vi "Variable@LInsert__Parameter.vi"(1 "ParamterIn":string) -> (0 "ParamterOut":string)   [LabVIEW 2019]
uses:
  <vilib>/regexp/Match Regular Expression.xnode
panel:
  in  "Pattern":string(combo)
  in  "Before/After":string(combo)
  in  "Section":string(combo)
  in  "Value":string(combo)
  in  "Variale":string(combo)
  in  "Confirm":bool
  # "Variable@LInsert $Variable,$Value,Before|After [value1,value2...](,$Section)"
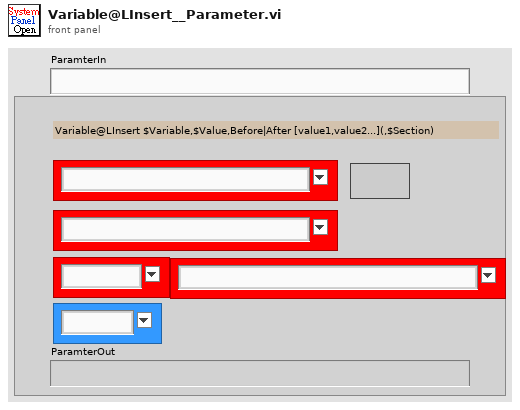
[diagram p1: front panel]
types:
  T1 = enum16{"Get", "Init", "Set", "Delete", "GetElement", "Inc", "Dec", "ReName"}
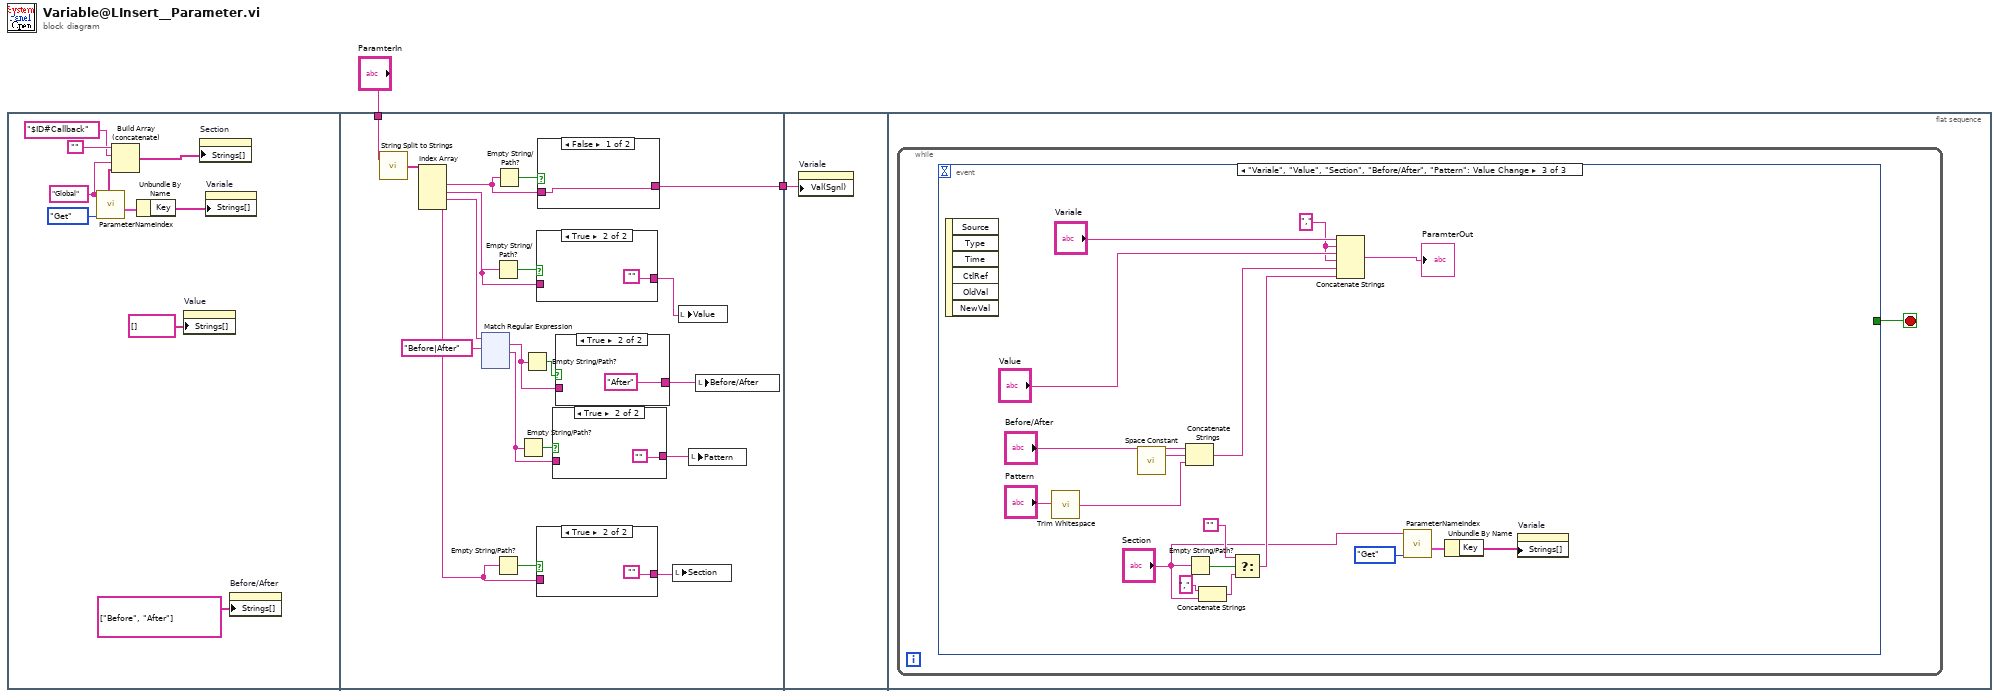
[diagram p0: block diagram]
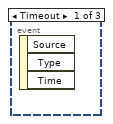
[diagram p7: hidden frame]
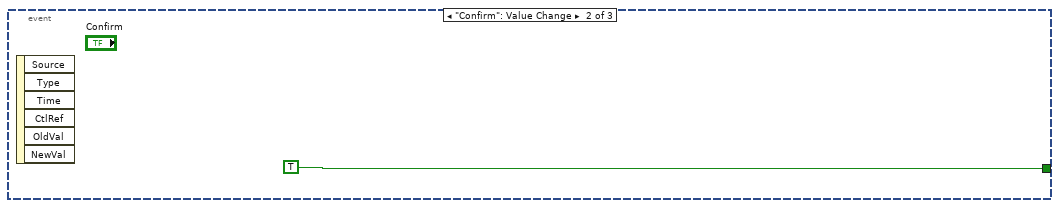
[diagram p8: hidden frame]
diagram:
  n1 = flat-sequence {
    tunnel: "ParamterIn" -> [w27]
    tunnel: [w29] -> w1
    tunnel: w1 -> [w156]
    frame #0 {
      w6 = "Global" ("VariableSection")
      n2 = call "ParameterNameIndex.vi"("OP"=T1."Get", "VariableSection"=w6) -> ("GlobalKeyValue"=w12:cluster{"Key":string[], "Value":string[]}, "SectionList"=w7:string[])  [unwired: 3 in, 5 out]
      n3 = Build Array (concatenate)("", "$ID#Callback" ("VariableSection"), w6, w7) -> (w4:string[])
      n4 = Unbundle By Name(w12) -> ("Key"=w11:string[])
      n5 = property on="Value" class="CmbBox"("Strings[]"=string[] [] ("Strings []")) -> ()  [unwired: 2 in, 2 out]
      n6 = property on="Section" class="CmbBox"("Strings[]"=w4) -> ()  [unwired: 2 in, 2 out]
      n7 = property on="Variale" class="CmbBox"("Strings[]"=w11) -> ()  [unwired: 2 in, 2 out]
      n8 = property on="Before/After" class="CmbBox"("Strings[]"=string[] ["Before", "After"] ("Strings []")) -> ()  [unwired: 2 in, 2 out]
    }
    frame #1 {
      n9 = call "String Split to Strings.vi"("String"=w27) -> ("Array"=w26:string[])  [unwired: 1 in]
      n10 = Index Array(array=w26) -> (element #1=w25:string, element #2=w24:string, element #3=w20:string, element #4=w21:string)  [unwired: 4 in]
      n11 = xnode "Match Regular Expression"("input string"=w20, "regular expression"="Before|After") -> ("whole match"=w18:string, "after match"=w14:string)  [unwired: 4 in, 3 out]
      n12 = Empty String/Path?(string/path=w24) -> (empty?=w30:bool)
      n13 = Empty String/Path?(string/path=w21) -> (empty?=w23:bool)
      n14 = Empty String/Path?(string/path=w25) -> (empty?=w31:bool)
      n15 = Empty String/Path?(string/path=w14) -> (empty?=w15:bool)
      n16 = Empty String/Path?(string/path=w18) -> (empty?=w17:bool)
      n17 = case shown="True" w30 {
        tunnel: w24 -> [w152 _]
        tunnel: [w152 ""] -> w28
        frame False {
        }
        frame True {
        }
      }
      n18 = case shown="True" w23 {
        tunnel: w21 -> [w150 _]
        tunnel: [w150 ""] -> w22
        frame False {
        }
        frame True {
        }
      }
      n19 = case shown="False" w31 {
        tunnel: w25 -> [w154 w155]
        tunnel: [w154 w155] -> w29
        frame False {
        }
        frame True {
        }
      }
      n20 = case shown="True" w15 {
        tunnel: w14 -> [w32 _]
        tunnel: [w32 ""] -> w13
        frame False {
        }
        frame True {
        }
      }
      n21 = case shown="True" w17 {
        tunnel: w18 -> [w34 _]
        tunnel: [w34 "After"] -> w16
        frame False {
        }
        frame True {
        }
      }
      n22 = local write "Section"(w22) -> ()
      n23 = local write "Value"(w28) -> ()
      n24 = local write "Pattern"(w13) -> ()
      n25 = local write "Before/After"(w16) -> ()
    }
    frame #2 {
      n26 = property on="Variale" class="CmbBox"("Val(Sgnl)"=w156) -> ()  [unwired: 2 in, 2 out]
    }
    frame #3 {
      n27 = while {
        stop <- w157 stop-if-true
        n28 = event shown="[2] \"Variale\", \"Value\", \"Section\", \"Before/After\", \"Pattern\": Value Change" {
          selector: _ -> [_ _ _]
          dyn-events: _ -> [_ _ _]
          timeout: _ -> [_ _ _]
          tunnel: [_ TRUE _] -> w157
          event Timeout {
            n29 = event-data() -> ()  [unwired: 1 in, 3 out]
          }
          event "Confirm": Value Change {
            n30 = event-data() -> ()  [unwired: 1 in, 6 out]
          }
          event "Variale", "Value", "Section", "Before/After", "Pattern": Value Change {
            w166 = "," ("string")
            n31 = event-data() -> ()  [unwired: 1 in, 6 out]
            n32 = call <vilib>:"Trim Whitespace.vi"("string"="Pattern") -> ("trimmed string"=w162:string)  [unwired: 1 in]
            n33 = call <vilib>:"Space Constant.vi"() -> ("String"=w167:string)
            n34 = Concatenate Strings("Before/After", w167, w162) -> (w165:string)
            n35 = Empty String/Path?(string/path="Section") -> (empty?=w172:bool)
            n36 = Concatenate Strings("," ("string"), "Section") -> (w173:string)
            n37 = Select(t="", s=w172, f=w173) -> (s? t:f=w164:string)
            n38 = Concatenate Strings("Variale", w166, "Value", w166, w165, w164) -> (→"ParamterOut":string)
            n39 = call "ParameterNameIndex.vi"("OP"=T1."Get", "VariableSection"="Section") -> ("GlobalKeyValue"=w160:cluster{"Key":string[], "Value":string[]})  [unwired: 3 in, 6 out]
            n40 = Unbundle By Name(w160) -> ("Key"=w171:string[])
            n41 = property on="Variale" class="CmbBox"("Strings[]"=w171) -> ()  [unwired: 2 in, 2 out]
          }
        }
      }
    }
  }
